vi "Amplitude_Calculation_for_finetuning.vi"(9 "Amplitude_In(V)":dbl=0.605 min=0.0 format="%.3f", 10 "Ist_Pegel(dBSPL)":dbl=94.02694316227692, 11 "Soll_Pegel(dBSPL)":i32=-1) -> (3 "Amplitude_Out(V)":dbl=0.605 min=0.0 format="%.3f")   [LabVIEW 2018]
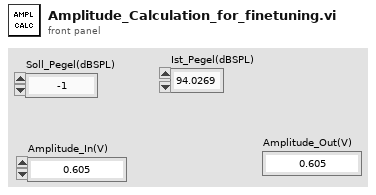
[diagram p1: front panel]
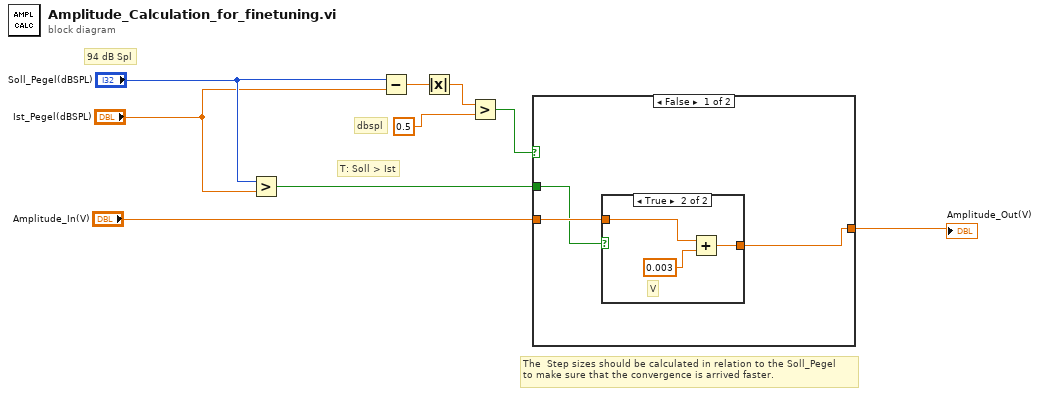
[diagram p0: block diagram]
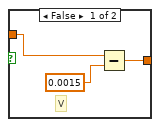
[diagram p2: hidden frame]
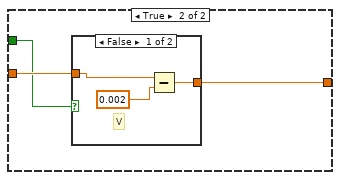
[diagram p3: hidden frame]
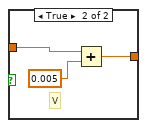
[diagram p4: hidden frame]
diagram:
  # "The  Step sizes should be calculated in relation to the Soll_Pegel\nto make sure that the convergence is arrived faster."
  # "T: Soll > Ist"
  # "94 dB Spl"
  # "dbspl"
  n1 = Greater?(x="Soll_Pegel(dBSPL)", y="Ist_Pegel(dBSPL)") -> (0:w1:bool)
  n2 = Subtract(x="Soll_Pegel(dBSPL)", y="Ist_Pegel(dBSPL)") -> (x-y=w9:dbl)
  n3 = Absolute Value(x=w9) -> (abs(x)=w8:dbl)
  n4 = Greater?(x=w8, y=0.5) -> (0:w6:bool)
  n5 = case shown="False" w6 {
    tunnel: "Amplitude_In(V)" -> [w12 w21]
    tunnel: [w11 w20] -> w4
    tunnel: w1 -> [w10 w19]
    frame False {
      n6 = case shown="True" w10 {
        tunnel: w12 -> [w13 w17]
        tunnel: [w14 w16] -> w11
        frame False {
          # "V"
          n7 = Subtract(x=w13, y=0.0015) -> (x-y=w14:dbl)
        }
        frame True {
          # "V"
          n8 = Add(x=w17, y=0.003) -> (x+y=w16:dbl)
        }
      }
    }
    frame True {
      n9 = case shown="False" w19 {
        tunnel: w21 -> [w23 w27]
        tunnel: [w22 w25] -> w20
        frame False {
          # "V"
          n10 = Subtract(x=w23, y=0.002) -> (x-y=w22:dbl)
        }
        frame True {
          # "V"
          n11 = Add(x=w27, y=0.005) -> (x+y=w25:dbl)
        }
      }
    }
  }
  "Amplitude_Out(V)" <- w4
